vi "String Indicator.vi"(10 "String Indicator":string, 11 "Ex Event Actor in":refnum<class "Ex Event Actor.lvclass">) -> (3 "Ex Event Actor out":refnum<class "Ex Event Actor.lvclass">)   [LabVIEW 2021, in "Ex Event Actor.lvlib" / "Ex Event Actor.lvclass"]
uses:
  Ex Event Actor.lvclass
  Ex Event Actor.lvclass/Ex Event Actor.ctl
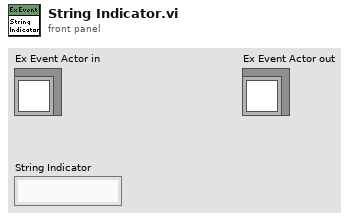
[diagram p1: front panel]
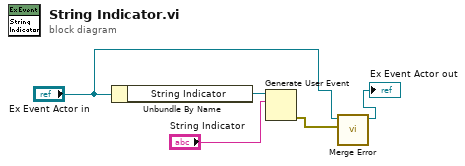
[diagram p0: block diagram]
diagram:
  n1 = Unbundle By Name("Ex Event Actor in") -> ("String Indicator"=w5:refnum<user-event>)
  n2 = Generate User Event(user event=w5, event data cluster="String Indicator") -> (error out=w3:errorcluster)  [unwired: 2 in, 1 out]
  n3 = call-dynamic "Merge Error.vi"("Error"=w3, "Ex Event Actor in"="Ex Event Actor in") -> ("Ex Event Actor out"=→"Ex Event Actor out":refnum<class "Ex Event Actor.lvclass">)  [unwired: 9 in]
